vi "LPC set speak rate.vi"(8 "error in (no error)":errorcluster, 10 "speak rate":dbl, 11 "VISA resource name":refnum<visa-resource-name>="GPIB0::8::INSTR") -> (0 "error out":errorcluster, 3 "VISA resource name out":refnum<visa-resource-name>)   [LabVIEW 2009, in "BEOC LPC.lvlib"]
doc: "Sets the speak rate of the LPC (laser power controller). This controls the rate at which the LPC sends back log entries. The speak rate should be set to zero while issuing commands or performing queries, to avoid reading a log entry when another response was expected."
uses:
  BEOC LPC.lvlib
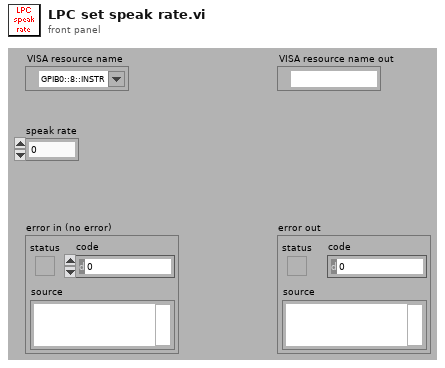
[diagram p1: front panel]
types:
  T1 = typedef "Semaphore RefNum" = refnum<k1>
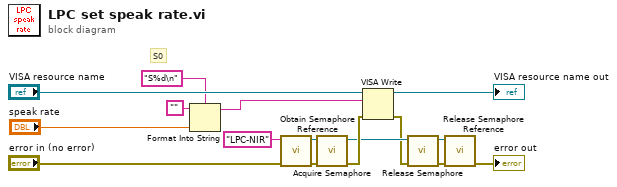
[diagram p0: block diagram]
diagram:
  # "S0"
  n1 = Format Into String(format string="S%d\n", initial string="", "speak rate") -> (resulting string=w12:string)  [unwired: 1 in, 1 out]
  n2 = call <vilib>:"Obtain Semaphore Reference.vi"("error in (no error)"="error in (no error)", "name (unnamed)"="LPC-NIR") -> ("error out"=w8:errorcluster, "semaphore"=w7:T1)  [unwired: 1 in, 3 out]
  n3 = call <vilib>:"Acquire Semaphore.vi"("error in (no error)"=w8, "semaphore"=w7) -> ("error out"=w4:errorcluster, "semaphore out"=w3:T1)  [unwired: 1 in, 3 out]
  n4 = VISA Write(VISA resource name="VISA resource name", write buffer=w12, error in (no error)=w4) -> (VISA resource name out=→"VISA resource name out":refnum<visa-resource-name>, error out=w2:errorcluster)  [unwired: 1 out]
  n5 = call <vilib>:"Release Semaphore.vi"("error in (no error)"=w2, "semaphore"=w3) -> ("error out"=w6:errorcluster, "semaphore out"=w5:T1)  [unwired: 4 out]
  n6 = call <vilib>:"Release Semaphore Reference.vi"("error in (no error)"=w6, "semaphore"=w5) -> ("error out"=→"error out":errorcluster)  [unwired: 9 out]
